vi "Print Error.vi"(5 "Custom Device? (T)":bool=TRUE, 7 "error out":errorcluster, 9 "Note (empty)":string, 10 "Your code's public name":string) -> ()   [LabVIEW 2023, in "PXIe-4139 Custom Device.lvlib"]
doc: "Prints error information out to the console. Provide your code's public name. For example, if your code is about J1939, put that here so the user knows what this printed error information has to do with.\n\nIf this is not a NI VeriStand custom device, write false to the Custom Device? input. This will change the error output.\n\nIf the 'note' field is empty, it is not printed to the console.\n\nExample output 1:\n******J1939 ERROR******\nSource: blah.vi\nCode: 535\n******J1939 ERROR******\n\nExample output 2:\n******XCP and CCP Master CUSTOM DEVICE ERROR******\nSource: blah.vi\nCode: 535\nUser Note: before write\n******XCP and CCP Master CUSTOM DEVICE ERROR******"
uses:
  PXIe-4139 Custom Device.lvlib
  <vilib>/NI VeriStand/Custom Device Tools/Custom Device Utility Library/Custom Device Utility Library.lvlib
  <vilib>/NI VeriStand/Custom Device Tools/Custom Device Utility Library/RT Debug String Color Spec.ctl
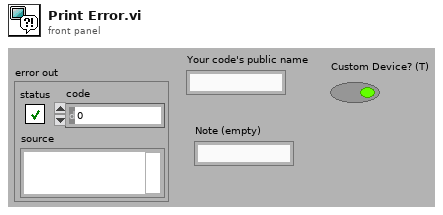
[diagram p1: front panel]
types:
  T1 = typedef "Custom Device Utility Library.lvlib/RT Debug String Color Spec.ctl" = u16
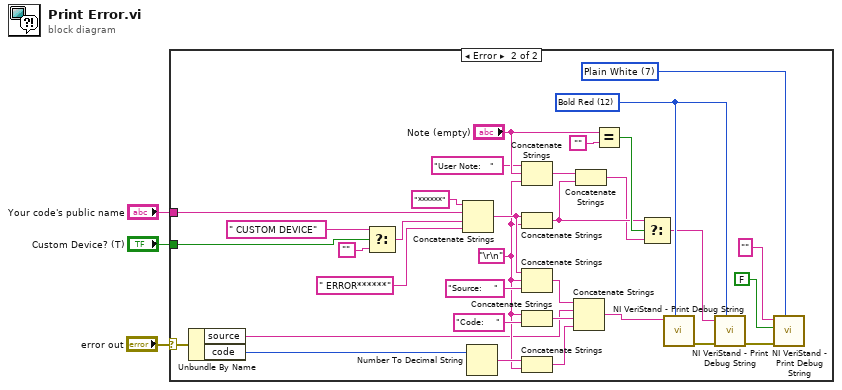
[diagram p0: block diagram]
diagram:
  n1 = case shown="Error" "error out" {
    selector: "error out" -> [_ w36]
    tunnel: "Custom Device? (T)" -> [_ w22]
    tunnel: "Your code's public name" -> [_ w15]
    frame No Error {
    }
    frame Error {
      w9 = T1 12 items=["Plain White"=7, "Bold White"=15, "Bold Blue"=9, "Bold Green"=10, "Bold Red"=12] ("Attribute")
      w18 = T1 7 items=["Plain White"=7, "Bold White"=15, "Bold Blue"=9, "Bold Green"=10, "Bold Red"=12] ("Attribute")
      w24 = "\r\n"
      n2 = Unbundle By Name(w36) -> ("source"=w14:string, "code"=w35:i32)
      n3 = Select(t=" CUSTOM DEVICE" ("String"), s=w22, f="") -> (s? t:f=w23:string)
      n4 = Concatenate Strings("******" ("String"), w15, w23, " ERROR******" ("String")) -> (w27:string)
      n5 = Number To Decimal String(number=w35) -> (decimal integer string=w32:string)  [unwired: 1 in]
      n6 = Concatenate Strings("User Note:   " ("string"), "Note (empty)", w24) -> (w5:string)
      n7 = Concatenate Strings(w27, w24) -> (w7:string)
      n8 = Concatenate Strings(w27, w24, "Source:    " ("String")) -> (w21:string)
      n9 = Concatenate Strings(w24, "Code:    " ("String")) -> (w17:string)
      n10 = Concatenate Strings(w32, w24) -> (w16:string)
      n11 = Concatenate Strings(w21, w14, w17, w16) -> (w12:string)
      n12 = Concatenate Strings(w5, w7) -> (w4:string)
      n13 = Equal?(x="Note (empty)", y="") -> (x = y?=w13:bool)
      n14 = Select(t=w7, s=w13, f=w4) -> (s? t:f=w8:string)
      n15 = call <vilib>:"NI VeriStand - Print Debug String.vi"("Attribute"=w9, "Message"=w12) -> ("error out"=w11:errorcluster)  [unwired: 9 in]
      n16 = call <vilib>:"NI VeriStand - Print Debug String.vi"("Attribute"=w9, "error in (no error)"=w11, "Message"=w8) -> ("error out"=w10:errorcluster)  [unwired: 8 in]
      n17 = call <vilib>:"NI VeriStand - Print Debug String.vi"("Attribute"=w18, "error in (no error)"=w10, "Add to log file? (F)"=FALSE ("Add to log file? (T)"), "Message"="") -> ()  [unwired: 7 in, 1 out]
    }
  }
